vi "READ_WRITE_I2C_EEPROM_24C01.vi"() -> ()   [LabVIEW 2017]
uses:
  libMPSSE.lvlib
panel:
  out "ID":u32
  out "Description":string
  out "Serial number":string
  out "sizeTransfered 2":u32
  out "buffer":string
  out "error out 2":errorcluster
  in  "Data to write 2":u8[](array[numeric])=[0]
  out "data string":string
  out "hex integer string":string[](array[string])
  out "sizeTransfered":u32
  in  "options read":T1={"Start bit"=TRUE, "Stop bit"=TRUE, "Acknowledge bit"=TRUE, "Reserved bit"=FALSE, "Multi byte I2C"=FALSE, "Multi bit I2C"=FALSE, "Ignore address"=FALSE, "Reserved bit 2"=FALSE}
  in  "Data to write":u8[](array[numeric])=[0, 0] format="%02x"
  in  "Config":T2={"ClockRate"=100000, "LatencyTimer"=1, "Disable 3 phase clocking"=FALSE, "Disable drive only 0"=FALSE} {"ClockRate" items=["I2C_CLOCK_STANDARD_MODE"=100000, "I2C_CLOCK_FAST_MODE"=400000, "I2C_CLOCK_FAST_MODE_PLUS"=1000000, "I2C_CLOCK_HIGH_SPEED_MODE"=3400000]}
  out "Data read":u8[](array[numeric]) format="%.0x"
  in  "options write":T1={"Start bit"=TRUE, "Stop bit"=FALSE, "Acknowledge bit"=TRUE, "Reserved bit"=FALSE, "Multi byte I2C"=FALSE, "Multi bit I2C"=FALSE, "Ignore address"=FALSE, "Reserved bit 2"=FALSE}
  in  "sizeToTransfer":u32=1
  in  "deviceAddress":u32=80 format="%.0b"
  out "numChannels out":u32
  out "error out":errorcluster
  # "This VI read an address of an EEPROM on I2C"
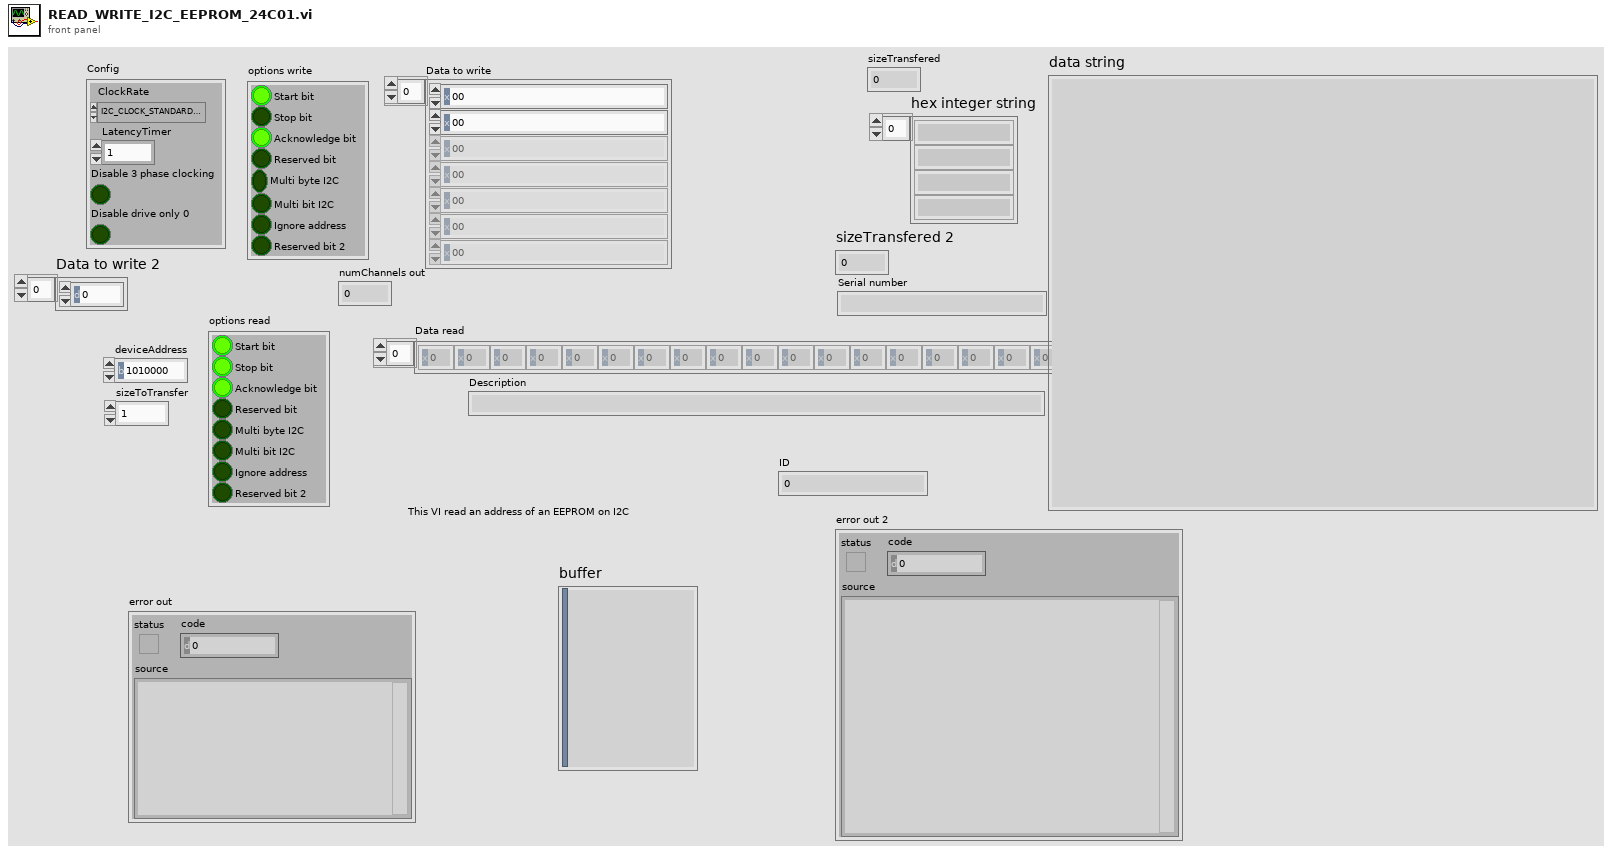
[diagram p1: front panel]
types:
  T1 = cluster{"Start bit":bool, "Stop bit":bool, "Acknowledge bit":bool, "Reserved bit":bool, "Multi byte I2C":bool, "Multi bit I2C":bool, "Ignore address":bool, "Reserved bit 2":bool}
  T2 = cluster{"ClockRate":u32, "LatencyTimer":u8, "Disable 3 phase clocking":bool, "Disable drive only 0":bool}
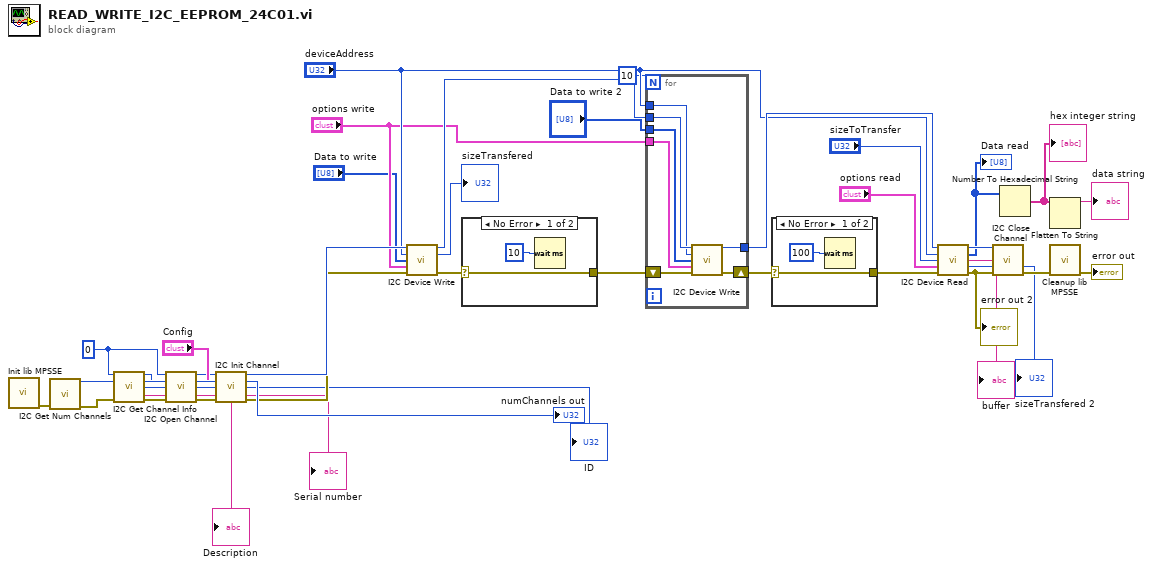
[diagram p0: block diagram]
diagram:
  w31 = u32 0 ("index")
  n1 = call "Init lib MPSSE.vi"() -> ("error out"=w37:errorcluster)  [unwired: 15 in]
  n2 = call "I2C Get Num Channels.vi"("error in (no error)"=w37) -> ("numChannels out"=→"numChannels out":u32, "error out"=w33:errorcluster)  [unwired: 13 in]
  n3 = call "I2C Get Channel Info.vi"("index"=w31, "error in (no error)"=w33) -> ("ftHandle"=w27:u32, "ID"=→"ID":u32, "Description"=→"Description":string, "Serial number"=→"Serial number":string, "error out"=w32:errorcluster)  [unwired: 6 in, 3 out]
  n4 = call "I2C Open Channel.vi"("handle"=w31, "index"=w27, "error in (no error)"=w32) -> ("handle out"=w29:u32, "error out"=w28:errorcluster)  [unwired: 11 in]
  n5 = call "I2C Init Channel.vi"("handle"=w29, "Config"="Config", "error in (no error)"=w28) -> ("handle out"=w25:u32, "error out"=w12:errorcluster)  [unwired: 11 in]
  n6 = call "I2C Device Write.vi"("handle"=w25, "deviceAddress"="deviceAddress", "Data to write"="Data to write", "options"="options write", "error in (no error)"=w12) -> ("handle out"=w18:u32, "sizeTransfered"=→"sizeTransfered":u32, "error out"=w7:errorcluster)  [unwired: 8 in]
  n7 = case shown="No Error" w7 {
    selector: w7 -> [w39 w40]
    tunnel: [w39 w40] -> w16
    frame No Error {
      n8 = Wait (ms)(milliseconds to wait=u32 10) -> ()  [unwired: 1 out]
    }
    frame Error {
    }
  }
  n9 = for {
    N: 10 -> [_]
    tunnel: w18 -> [w47]
    tunnel: [w46] -> w17
    tunnel: "deviceAddress" -> [w44]
    tunnel: "Data to write 2" -> [w43]
    tunnel: "options write" -> [w42]
    shift-right: [w41] -> w11
    shift-left: w16 -> [w45]
    n10 = call "I2C Device Write.vi"("handle"=w47, "deviceAddress"=w44, "Data to write"=w43, "options"=w42, "error in (no error)"=w45) -> ("handle out"=w46:u32, "error out"=w41:errorcluster)  [unwired: 8 in, 1 out]
  }
  n11 = case shown="No Error" w11 {
    selector: w11 -> [w49 w50]
    tunnel: [w49 w50] -> w10
    frame No Error {
      n12 = Wait (ms)(milliseconds to wait=u32 100) -> ()  [unwired: 1 out]
    }
    frame Error {
    }
  }
  n13 = call "I2C Device Read.vi"("handle"=w17, "Slave device address"="deviceAddress", "Size to transfer"="sizeToTransfer", "options"="options read", "error in (no error)"=w10) -> ("handle out"=w23:u32, "Data read"=w21:u8[], "buffer"=→"buffer":string, "sizeTransfered"=→"sizeTransfered 2":u32, "error out"=w24:errorcluster)  [unwired: 6 in]
  "Data read" <- w21
  "error out 2" <- w24
  n14 = call "I2C Close Channel.vi"("handle"=w23, "error in (no error)"=w24) -> ("error out"=w34:errorcluster)  [unwired: 13 in]
  n15 = Number To Hexadecimal String(2:w21) -> (0:w20:string[])  [unwired: 1 in]
  "hex integer string" <- w20
  n16 = Flatten To String(anything=w20) -> (data string=→"data string":string)  [unwired: 3 in, 2 out]
  n17 = call "Cleanup lib MPSSE.vi"("error in (no error)"=w34) -> ("error out"=→"error out":errorcluster)  [unwired: 14 in]
